vi "Update Drawing.vi"(8 "error in (no error)":errorcluster, 10 "Field Drawing":picture, 11 "Vision in":refnum<class "Vision.lvclass">) -> (0 "error out":errorcluster, 3 "Vision out":refnum<class "Vision.lvclass">)   [LabVIEW 2022 SP3, in "Vision.lvlib" / "Vision.lvclass"]
uses:
  Vision.lvclass
  Vision.lvclass/Vision.ctl
  <vilib>/ActorFramework/Actor/Actor.lvclass
  Phoenix/Phoenix Messages/Update Drawing Msg/Update Drawing Msg.lvclass
  C:/Program Files (x86)/National Instruments/LabVIEW 2022/vi.lib/MGI/Monitored Actor/Monitored Actor/Monitored Actor/Monitored Actor.lvclass
  C:/Program Files (x86)/National Instruments/LabVIEW 2022/vi.lib/ActorFramework/Actor/Actor.lvclass
  C:/Users/ebert/Documents/codes/SSL/repo/Phoenix Reborn/Vision/Vision/Vision.lvclass
  C:/Users/ebert/Documents/codes/SSL/repo/Phoenix Reborn/UDP Data Receiver/UDP Data Receiver/UDP Data Receiver.lvclass
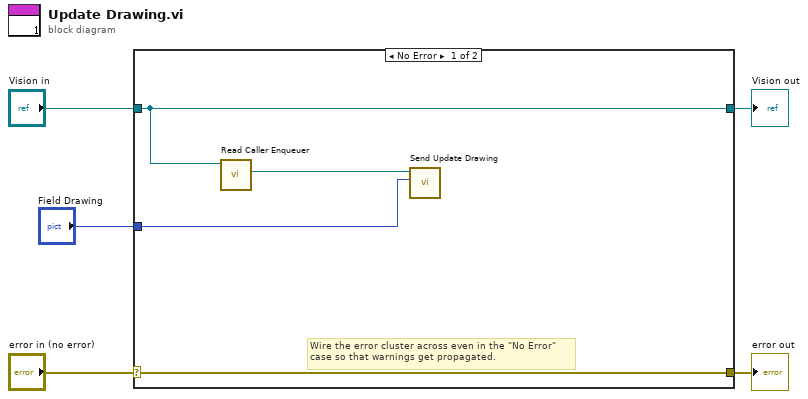
[diagram p0: block diagram]
diagram:
  n1 = case shown="No Error" "error in (no error)" {
    selector: "error in (no error)" -> [w9 w11]
    tunnel: [w9 w11] -> w4
    tunnel: [w8 w10] -> w2
    tunnel: "Vision in" -> [w8 w10]
    tunnel: "Field Drawing" -> [w6 _]
    frame No Error {
      # "Wire the error cluster across even in the \"No Error\"\ncase so that warnings get propagated."
      n2 = call <vilib>:"Read Caller Enqueuer.vi"("Actor"=w8) -> ("Caller Enqueuer"=w7:refnum<class "Message Enqueuer.lvclass">)  [unwired: 10 in]
      n3 = call "Send Update Drawing.vi"("Field Drawing"=w6, "Message Enqueuer"=w7) -> ()  [unwired: 8 in, 2 out]
    }
    frame Error {
    }
  }
  "error out" <- w4
  "Vision out" <- w2
